vi "ReadScript.vi"(8 "error in (no error)":errorcluster, 11 "String":string) -> (0 "error out":errorcluster, 3 "all rows":string[][](array[string]))   [LabVIEW 2019, in "Scripts.lvclass"]
uses:
  Scripts.lvclass
  <vilib>/Utility/file.llb/Read Delimited Spreadsheet (string).vi
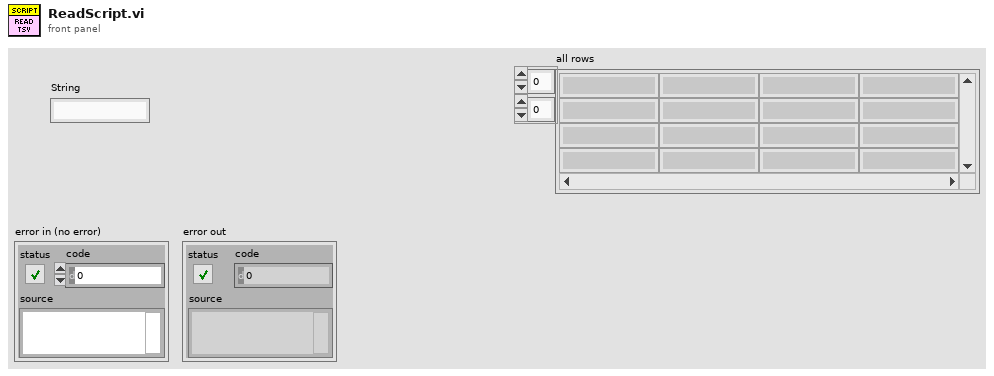
[diagram p1: front panel]
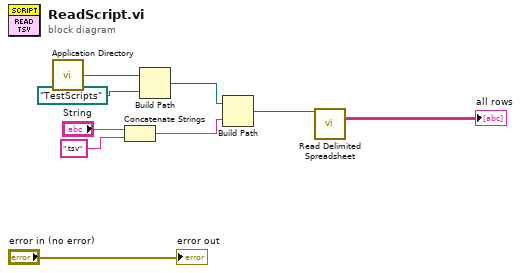
[diagram p0: block diagram]
diagram:
  n1 = call <vilib>:"Application Directory.vi"() -> ("Application Directory"=w7:path)
  n2 = Concatenate Strings("String", ".tsv" ("string")) -> (w4:string)
  n3 = Build Path(base path=w7, name or relative path=path "TestScripts") -> (appended path=w5:path)
  n4 = Build Path(base path=w5, name or relative path=w4) -> (appended path=w3:path)
  n5 = call-poly <vilib>:"Read Delimited Spreadsheet.vi"("file path (dialog if empty)"=w3) -> ("all rows"=→"all rows":string[][])  [unwired: 9 in, 5 out]
  "error out" <- "error in (no error)"
